vi "Where.vi"(7 "Where/And":string(combo)="and", 8 "error in (no error)":errorcluster, 9 "ColumnData Array":string[](array[string]), 10 "ColumnName Array":string[](array[string]), 11 "DataBase_SQL in":refnum<class "DataBase_SQL.lvclass">) -> (0 "error out":errorcluster, 2 "String":string, 3 "DataBase_SQL out":refnum<class "DataBase_SQL.lvclass">, 4 "ColumnData Array Out":string[](array[string]), 5 "ColumnName Array Out":string[](array[string]))   [LabVIEW 2021, in "DataBase_SQL.lvclass"]
uses:
  <userlib>/John_Lib/DataBase/DataBase_SQL/DataBase_SQL.lvclass
  <userlib>/John_Lib/DataBase/DataBase_SQL/DataBase_SQL.lvclass/DataBase_SQL.ctl
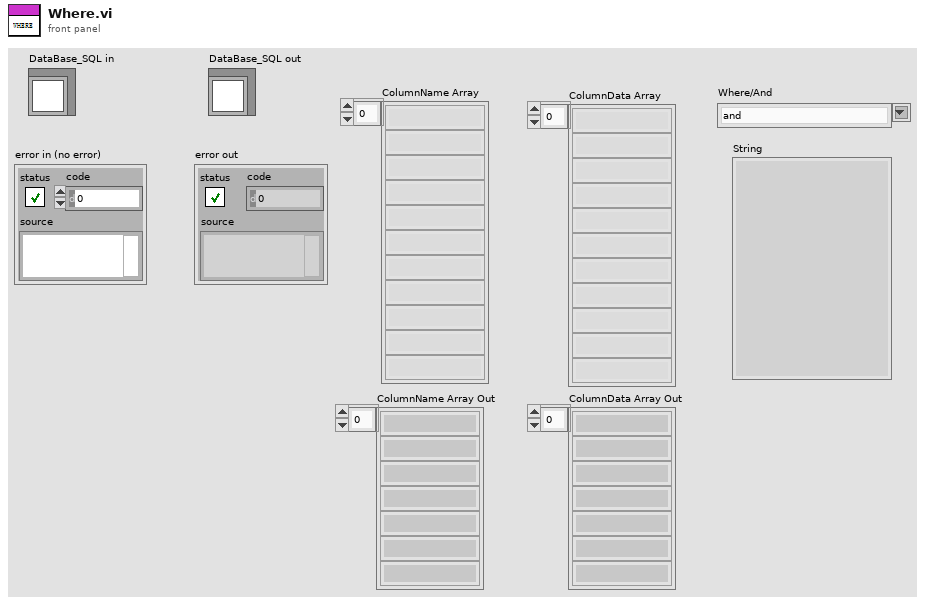
[diagram p1: front panel]
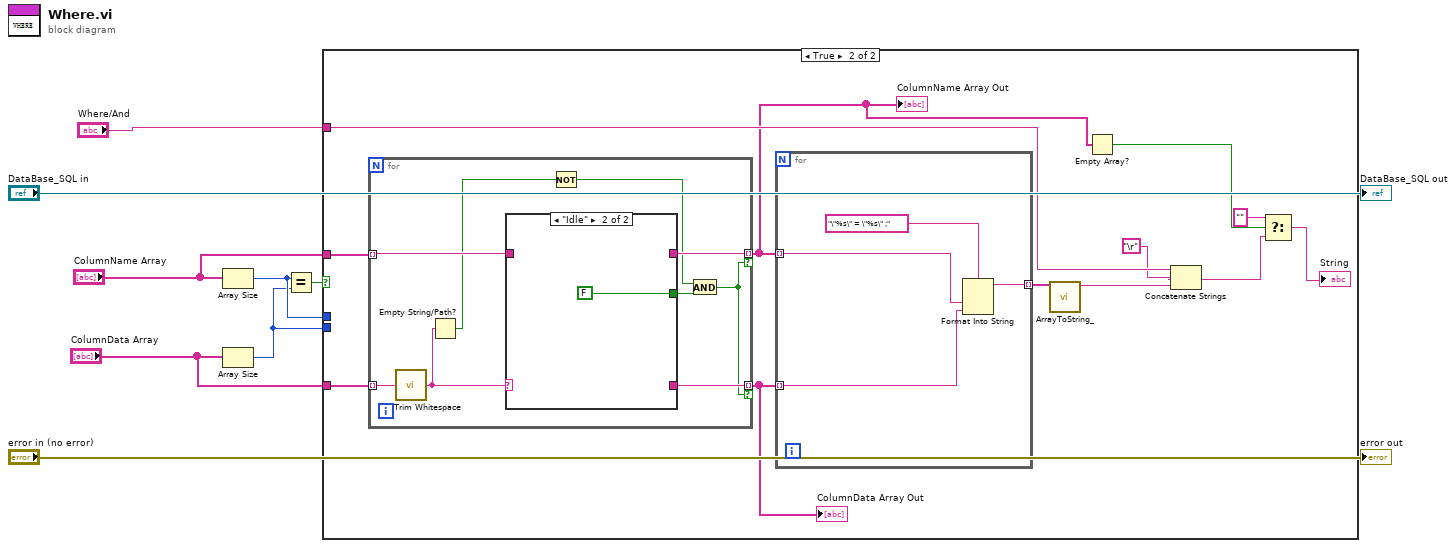
[diagram p0: block diagram]
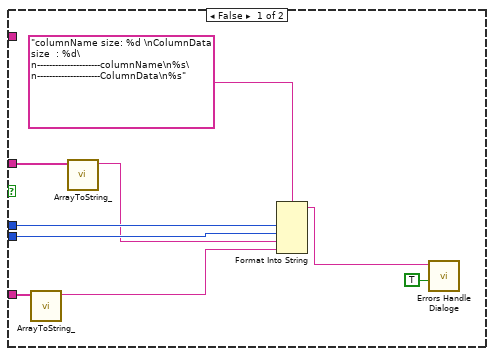
[diagram p2: hidden frame]
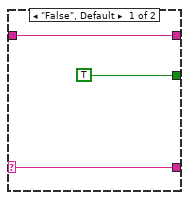
[diagram p3: hidden frame]
diagram:
  n1 = Array Size(array="ColumnName Array") -> (size(s)=w3:i32)
  n2 = Array Size(array="ColumnData Array") -> (size(s)=w2:i32)
  n3 = Equal?(x=w3, y=w2) -> (x = y?=w6:bool)
  n4 = case shown="True" w6 {
    tunnel: "ColumnName Array" -> [w15 w28]
    tunnel: "ColumnData Array" -> [w14 w29]
    tunnel: w3 -> [w13 _]
    tunnel: w2 -> [w12 _]
    tunnel: "Where/And" -> [_ w24]
    frame False {
      n5 = call <userlib>:"ArrayToString_.vi"("Array"=w14) -> ("String"=w10:string)  [unwired: 10 in]
      n6 = call <userlib>:"ArrayToString_.vi"("Array"=w15) -> ("String"=w11:string)  [unwired: 10 in]
      n7 = Format Into String(format string="columnName size: %d \nColumnData size  : %d\n---------------------columnName\n%s\n---------------------ColumnData\n%s", w13, w12, w11, w10) -> (resulting string=w9:string)  [unwired: 2 in, 1 out]
      n8 = call <userlib>:"Errors Handle Dialoge.vi"("DisplayDialog"=TRUE, "Message"=w9) -> ()  [unwired: 8 in, 2 out]
    }
    frame True {
      n9 = for {
        tunnel: w29 -> [w42] mode=indexing
        tunnel: w28 -> [w38] mode=indexing
        tunnel: [w40] -> w27 mode=indexing if=w36
        tunnel: [w39] -> w22 mode=indexing if=w36
        n10 = call <vilib>:"Trim Whitespace.vi"("string"=w42) -> ("trimmed string"=w41:string)  [unwired: 1 in]
        n11 = Empty String/Path?(string/path=w41) -> (empty?=w35:bool)
        n12 = case shown="\"Idle\"" w41 {
          selector: w41 -> [w44 _]
          tunnel: [w45 _] -> w39
          tunnel: w38 -> [w45 _]
          tunnel: [w44 _] -> w40
          tunnel: [TRUE FALSE] -> w37
          frame "False", Default {
          }
          frame "Idle" {
          }
        }
        n13 = Not(x=w35) -> (.not. x?=w34:bool)
        n14 = And(x=w34, y=w37) -> (x .and. y?=w36:bool)
      }
      "ColumnName Array Out" <- w22
      "ColumnData Array Out" <- w27
      n15 = for {
        tunnel: w22 -> [w32] mode=indexing
        tunnel: w27 -> [w31] mode=indexing
        tunnel: [w30] -> w26 mode=indexing
        n16 = Format Into String(format string="\"%s\" = \"%s\" ;", w32, w31) -> (resulting string=w30:string)  [unwired: 2 in, 1 out]
      }
      n17 = call <userlib>:"ArrayToString_.vi"("Array"=w26) -> ("String"=w25:string)  [unwired: 10 in]
      n18 = Empty Array?(array=w22) -> (empty?=w21:bool)
      n19 = Concatenate Strings(w24, "\r", w25) -> (w19:string)
      n20 = Select(t="", s=w21, f=w19) -> (s? t:f=→"String":string)
    }
  }
  "error out" <- "error in (no error)"
  "DataBase_SQL out" <- "DataBase_SQL in"
